vi "Init.vi"(0 "serial port":T1=enum."MXP TTL", 5 "baud rate":u32=19200, 11 "error in":errorcluster) -> (4 "comm interface out":refnum<class "Pixy Com.lvclass">, 15 "error out":errorcluster)   [LabVIEW 2018, in "RoboRIO UART.lvclass"]
doc: "Initializes a Pixy2 communication session for the RoboRIO UART bus."
uses:
  RoboRIO UART.lvclass
  library/Interface/Pixy Com.lvclass
  <vilib>/Rock Robotics/WPI/SerialPort/WPI_SerialPort.ctl
  C:/Users/David/Documents/GitHub/Pixy2LabVIEW/source/library/Interface/Pixy Com.lvclass
  RoboRIO UART.lvclass/RoboRIO UART.ctl
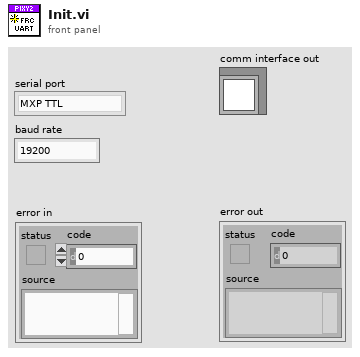
[diagram p1: front panel]
types:
  T1 = typedef "WPI_SerialPort.ctl" = enum16{"Onboard RS-232", "MXP TTL", "USB 1", "USB 2"}
  T2 = typedef "WPI_SerialPortRef.ctl" = cluster{"DevStatus":errorcluster, "Serial Port Name":refnum<visa-resource-name>}
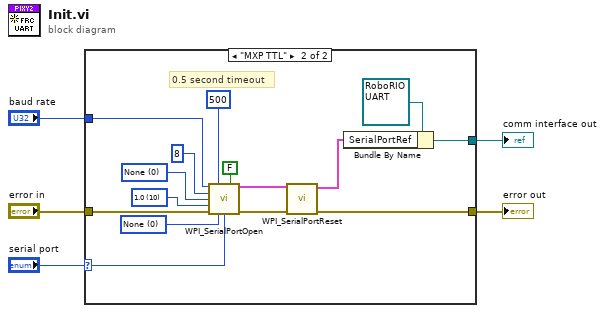
[diagram p0: block diagram]
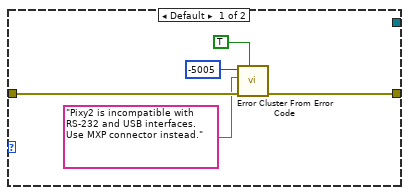
[diagram p2: hidden frame]
diagram:
  n1 = case shown="\"MXP TTL\"" "serial port" {
    selector: "serial port" -> [_ w22]
    tunnel: "error in" -> [w10 w25]
    tunnel: "baud rate" -> [_ w24]
    tunnel: [_ w15] -> w2
    tunnel: [w9 w12] -> w1
    frame Default {
      n2 = call <vilib>:"Error Cluster From Error Code.vi"("show call chain? (False)"=TRUE, "error in (no error)"=w10, "error message (\"\")"="Pixy2 is incompatible with RS-232 and USB interfaces. Use MXP connector instead." ("error message (\"\")"), "error code (0)"=-5005) -> ("error out"=w9:errorcluster)  [unwired: 5 in]
    }
    frame "MXP TTL" {
      w17 = u16 0 items=["None", "Odd", "Even", "Mark", "Space"] ("Parity")
      w21 = u16 10 items=["1.0"=10, "1.5"=15, "2.0"=20] ("Stop Bits")
      w23 = u16 0 items=["None", "XON/XOFF", "RTS/CTS", "XON/XOFF & RTS/CTS", "DTR/DSR", "XON/XOFF & DTR/DSR"] ("Flow Control")
      # "0.5 second timeout"
      n3 = call <vilib>:"WPI_SerialPortOpen.vi"("Baud Rate"=w24, "Timeout Value (ms)"=u32 500, "Enable Termination Char? (T)"=FALSE, "Data Bits"=u16 8, "Parity"=w17, "Stop Bits"=w21, "error in (no error)"=w25, "Flow Control"=w23, "Serial Port"=w22) -> ("SerialPortRef"=w14:T2, "error out"=w13:errorcluster)  [unwired: 5 in]
      n4 = call <vilib>:"WPI_SerialPortReset.vi"("error in (no error)"=w13, "SerialPortRef"=w14) -> ("error out"=w12:errorcluster, "SerialPortRef"=w11:T2)  [unwired: 8 in]
      n5 = Bundle By Name(cluster=refnum<class "RoboRIO UART.lvclass"> refnum ("RoboRIO UART.lvclass"), "SerialPortRef"=w11) -> (w15:refnum<class "RoboRIO UART.lvclass">)
    }
  }
  "comm interface out" <- w2
  "error out" <- w1
